vi "test_cycles_per_sample.vi"(6 "initial delay":i32=7, 8 "cycles per sample":i32, 11 "index":i32) -> (0 "valid out":bool, 3 "array index":i32)   [LabVIEW 2013]
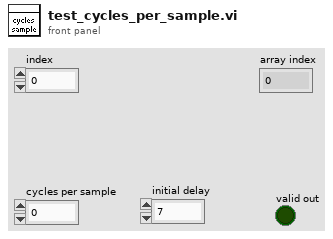
[diagram p1: front panel]
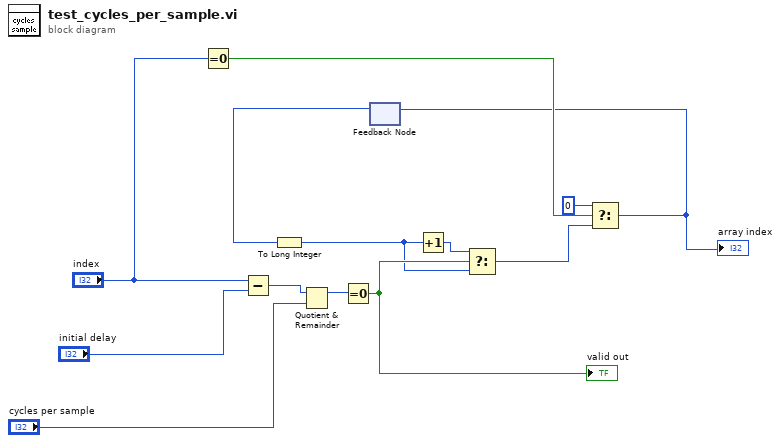
[diagram p0: block diagram]
diagram:
  n1 = Equal To 0?(x="index") -> (x = 0?=w4:bool)
  n2 = Subtract(x="index", y="initial delay") -> (x-y=w10:i32)
  n3 = Quotient & Remainder(x=w10, y="cycles per sample") -> (x-y*floor(x/y)=w13:i32)  [unwired: 1 out]
  n4 = Equal To 0?(x=w13) -> (x = 0?=w9:bool)
  "valid out" <- w9
  n5 = feedback #1() -> (w7:i32)  [unwired: 1 in]
  n6 = To Long Integer(number=w7) -> (32bit integer=w6:i32)
  n7 = Increment(x=w6) -> (x+1=w12:i32)
  n8 = Select(t=w12, s=w9, f=w6) -> (s? t:f=w3:i32)
  n9 = Select(t=0, s=w4, f=w3) -> (s? t:f=w1:i32)
  "array index" <- w1
  n10 = feedback-in #1(w1) -> ()
